vi "DAQmx.Dark.Current.test.-.Jason1.vi"() -> ()   [LabVIEW 2020]
uses:
  <vilib>/DAQmx/write.llb/DAQmx Write (Digital U32 1Chan 1Samp).vi
  <vilib>/DAQmx/write.llb/DAQmx Write (Digital Bool 1Line 1Point).vi
  <vilib>/DAQmx/create/channels.llb/DAQmx Create Channel (DO-Digital Output).vi
  <vilib>/DAQmx/miscellaneous.llb/DAQmx Fill In Error Info.vi
panel:
  in  "Data Pin 2":tag="Dev1/port0/line0:7"
  in  "Write Pin 2":tag="Dev1/port0/line0:7"
  in  "Data to Send 2":u32[](array[numeric])=[1, 2, 4, 8, 16, 32, 64, 128]
  in  "Clear Pin 2":tag="Dev1/port0/line0:7"
  in  "Sync Pin 2":tag="Dev1/port0/line0:7"
  in  "Clear Pin":tag="Dev1/port0/line0:7"
  in  "Sync Pin":tag="Dev1/port0/line0:7"
  in  "Data Pin":tag="Dev1/port0/line0:7"
  in  "Write Pin":tag="Dev1/port0/line0:7"
  in  "Data to Send":u32[](array[numeric])=[1, 2, 4, 8, 16, 32, 64, 128]
  # "This 8 bit signal will \nturn on 2 tubes. However,\nwe need to pad it with \n24 zeroes for it to work with\nDravin's circuit board. We\nwill always be sending 32\nbits at a time."
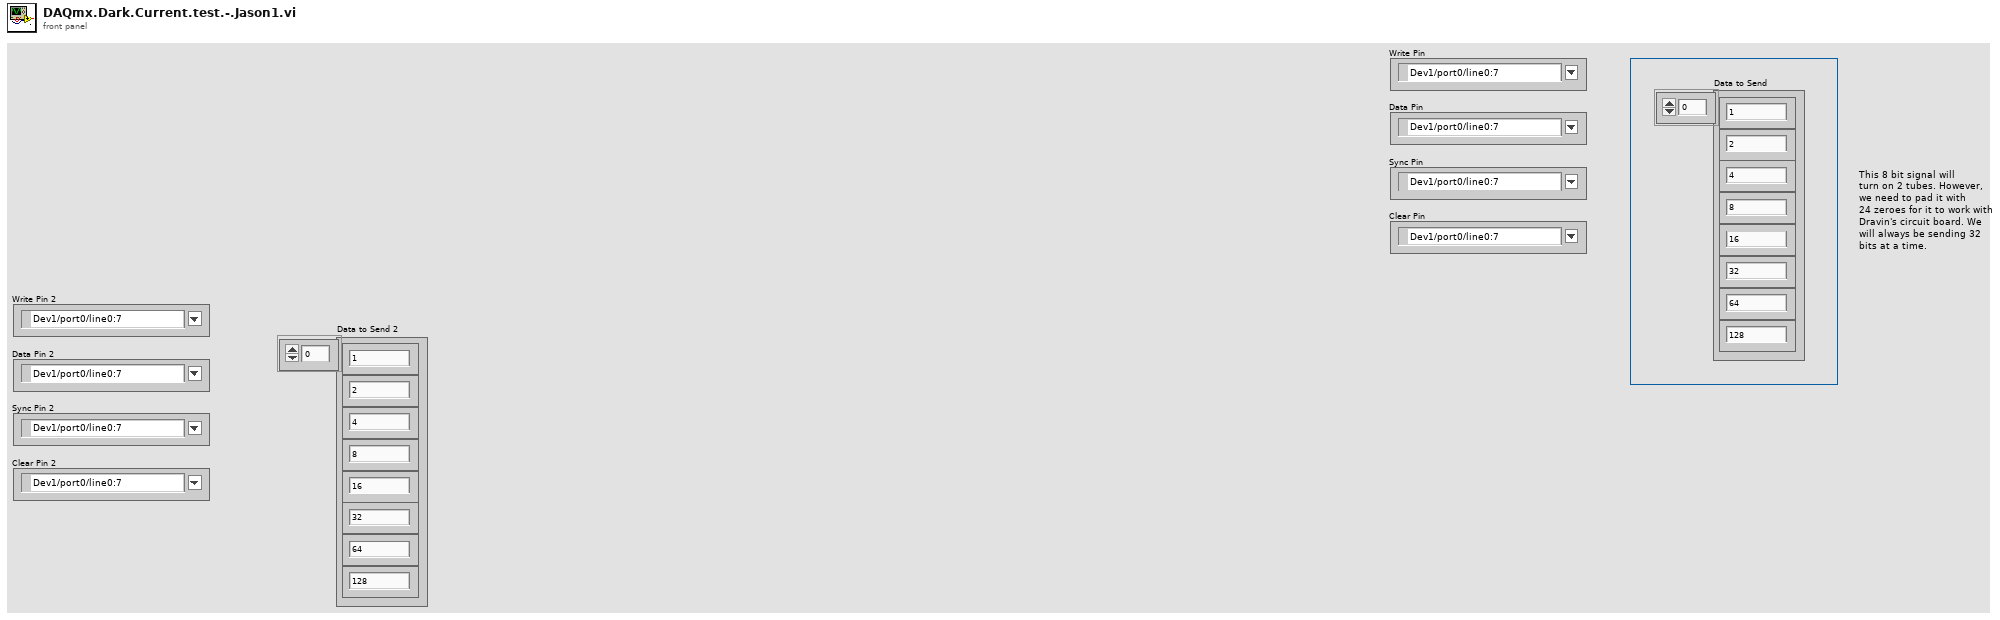
[diagram p1: front panel]
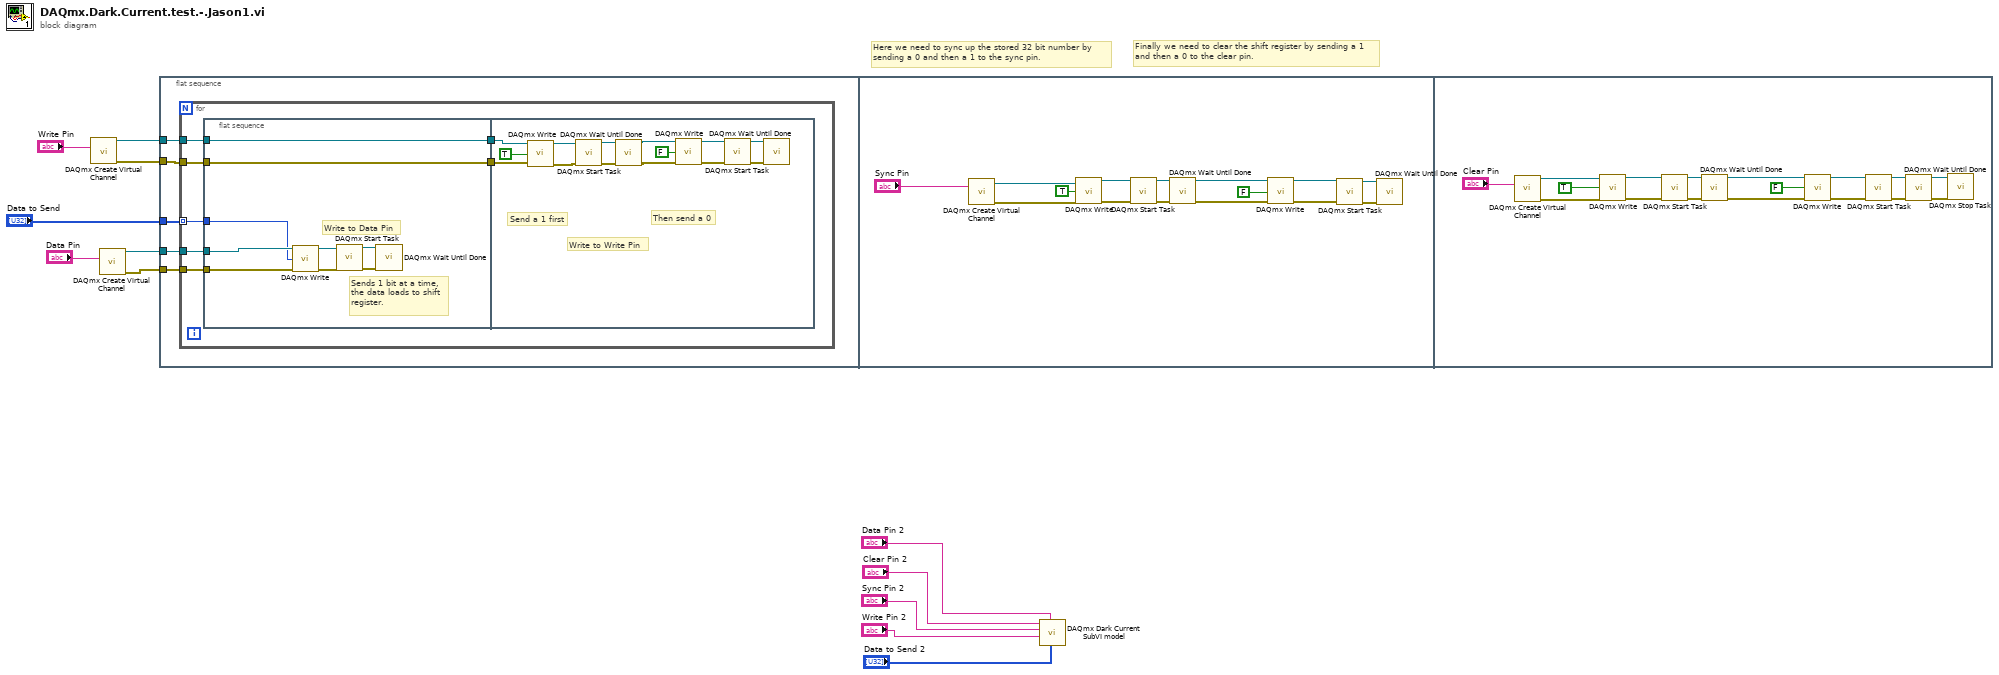
[diagram p0: block diagram]
diagram:
  # "Finally we need to clear the shift register by sending a 1\nand then a 0 to the clear pin."
  # "Here we need to sync up the stored 32 bit number by \nsending a 0 and then a 1 to the sync pin."
  n1 = call-poly <vilib>:"DAQmx Create Virtual Channel.vi"("lines"="Write Pin") -> ("task out"=w11:refnum<k21>, "error out"=w10:errorcluster)  [unwired: 13 in]
  n2 = call-poly <vilib>:"DAQmx Create Virtual Channel.vi"("lines"="Data Pin") -> ("task out"=w8:refnum<k21>, "error out"=w7:errorcluster)  [unwired: 13 in]
  n3 = flat-sequence {
    tunnel: w11 -> [w17]
    tunnel: w10 -> [w16]
    tunnel: w8 -> [w15]
    tunnel: w7 -> [w14]
    tunnel: "Data to Send" -> [w13]
    frame #0 {
      n4 = for {
        tunnel: w17 -> [w24]
        tunnel: w16 -> [w22]
        tunnel: w15 -> [w20]
        tunnel: w14 -> [w19]
        tunnel: w13 -> [w18] mode=indexing
        n5 = flat-sequence {
          tunnel: w24 -> [w33]
          tunnel: [w33] -> w23
          tunnel: w22 -> [w32]
          tunnel: [w32] -> w21
          tunnel: w20 -> [w31]
          tunnel: w19 -> [w30]
          tunnel: w18 -> [w29]
          tunnel: w23 -> [w35]
          tunnel: w21 -> [w34]
          frame #0 {
            # "Sends 1 bit at a time,\nthe data loads to shift\nregister."
            # "Write to Data Pin"
            n6 = call-poly <vilib>:"DAQmx Write.vi"("task/channels in"=w31, "data"=w29, "error in"=w30) -> ("task out"=w27:refnum<k21>, "error out"=w26:errorcluster)  [unwired: 10 in, 1 out]
            n7 = call <vilib>:"DAQmx Start Task.vi"("task/channels in"=w27, "error in"=w26) -> ("task out"=w25:refnum<k21>, "error out"=w28:errorcluster)  [unwired: 12 in]
            n8 = call <vilib>:"DAQmx Wait Until Done.vi"("task/channels in"=w25, "error in"=w28) -> ()  [unwired: 12 in, 2 out]
          }
          frame #1 {
            # "Then send a 0"
            # "Send a 1 first"
            # "Write to Write Pin"
            n9 = call-poly <vilib>:"DAQmx Write.vi"("task/channels in"=w35, "data"=TRUE, "error in"=w34) -> ("task out"=w46:refnum<k21>, "error out"=w45:errorcluster)  [unwired: 10 in, 1 out]
            n10 = call <vilib>:"DAQmx Start Task.vi"("task/channels in"=w46, "error in"=w45) -> ("task out"=w44:refnum<k21>, "error out"=w47:errorcluster)  [unwired: 12 in]
            n11 = call <vilib>:"DAQmx Wait Until Done.vi"("task/channels in"=w44, "error in"=w47) -> ("task out"=w37:refnum<k21>, "error out"=w36:errorcluster)  [unwired: 12 in]
            n12 = call-poly <vilib>:"DAQmx Write.vi"("task/channels in"=w37, "data"=FALSE, "error in"=w36) -> ("task out"=w39:refnum<k21>, "error out"=w38:errorcluster)  [unwired: 10 in, 1 out]
            n13 = call <vilib>:"DAQmx Start Task.vi"("task/channels in"=w39, "error in"=w38) -> ("task out"=w40:refnum<k21>, "error out"=w41:errorcluster)  [unwired: 12 in]
            n14 = call <vilib>:"DAQmx Wait Until Done.vi"("task/channels in"=w40, "error in"=w41) -> ()  [unwired: 12 in, 2 out]
          }
        }
      }
    }
    frame #1 {
      n15 = call-poly <vilib>:"DAQmx Create Virtual Channel.vi"("lines"="Sync Pin") -> ("task out"=w61:refnum<k21>, "error out"=w57:errorcluster)  [unwired: 13 in]
      n16 = call-poly <vilib>:"DAQmx Write.vi"("task/channels in"=w61, "data"=TRUE, "error in"=w57) -> ("task out"=w58:refnum<k21>, "error out"=w56:errorcluster)  [unwired: 10 in, 1 out]
      n17 = call <vilib>:"DAQmx Start Task.vi"("task/channels in"=w58, "error in"=w56) -> ("task out"=w59:refnum<k21>, "error out"=w55:errorcluster)  [unwired: 12 in]
      n18 = call <vilib>:"DAQmx Wait Until Done.vi"("task/channels in"=w59, "error in"=w55) -> ("task out"=w53:refnum<k21>, "error out"=w52:errorcluster)  [unwired: 12 in]
      n19 = call-poly <vilib>:"DAQmx Write.vi"("task/channels in"=w53, "data"=FALSE, "error in"=w52) -> ("task out"=w49:refnum<k21>, "error out"=w48:errorcluster)  [unwired: 10 in, 1 out]
      n20 = call <vilib>:"DAQmx Start Task.vi"("task/channels in"=w49, "error in"=w48) -> ("task out"=w51:refnum<k21>, "error out"=w50:errorcluster)  [unwired: 12 in]
      n21 = call <vilib>:"DAQmx Wait Until Done.vi"("task/channels in"=w51, "error in"=w50) -> ()  [unwired: 12 in, 2 out]
    }
    frame #2 {
      n22 = call-poly <vilib>:"DAQmx Create Virtual Channel.vi"("lines"="Clear Pin") -> ("task out"=w73:refnum<k21>, "error out"=w74:errorcluster)  [unwired: 13 in]
      n23 = call-poly <vilib>:"DAQmx Write.vi"("task/channels in"=w73, "data"=TRUE, "error in"=w74) -> ("task out"=w77:refnum<k21>, "error out"=w76:errorcluster)  [unwired: 10 in, 1 out]
      n24 = call <vilib>:"DAQmx Start Task.vi"("task/channels in"=w77, "error in"=w76) -> ("task out"=w79:refnum<k21>, "error out"=w78:errorcluster)  [unwired: 12 in]
      n25 = call <vilib>:"DAQmx Wait Until Done.vi"("task/channels in"=w79, "error in"=w78) -> ("task out"=w71:refnum<k21>, "error out"=w70:errorcluster)  [unwired: 12 in]
      n26 = call-poly <vilib>:"DAQmx Write.vi"("task/channels in"=w71, "data"=FALSE, "error in"=w70) -> ("task out"=w66:refnum<k21>, "error out"=w65:errorcluster)  [unwired: 10 in, 1 out]
      n27 = call <vilib>:"DAQmx Start Task.vi"("task/channels in"=w66, "error in"=w65) -> ("task out"=w68:refnum<k21>, "error out"=w67:errorcluster)  [unwired: 12 in]
      n28 = call <vilib>:"DAQmx Wait Until Done.vi"("task/channels in"=w68, "error in"=w67) -> ("task out"=w64:refnum<k21>, "error out"=w63:errorcluster)  [unwired: 12 in]
      n29 = call <vilib>:"DAQmx Stop Task.vi"("task/channels in"=w64, "error in"=w63) -> ()  [unwired: 12 in, 2 out]
    }
  }
  n30 = call "DAQmx Dark Current SubVI model.vi"("Data to Send in"="Data to Send 2", "Data Pin in"="Data Pin 2", "Write Pin in"="Write Pin 2", "Sync Pin in"="Sync Pin 2", "Clear Pin in"="Clear Pin 2") -> ()  [unwired: 7 in]
